vi "rad_Read FPGA Properties from INI.vi"(7 "section":string, 8 "error in (no error)":errorcluster, 11 "refnum in":T3) -> (0 "error out":errorcluster, 2 "FPGA Properties":T1=[{"Resource Name"=" ", "Path"=path ""}], 3 "refnum out":T3)   [LabVIEW 2013]
uses:
  <vilib>/Utility/config.llb/Config Data RefNum.ctl
  TypeDefs/rad_FPGA Properties.ctl
  TypeDefs/rad_FPGA Flash Properties.ctl
  <vilib>/Utility/config.llb/Read Key (I32).vi
  <vilib>/Utility/config.llb/Read Key (String).vi
  <vilib>/Utility/config.llb/NI_LVConfig.lvlib
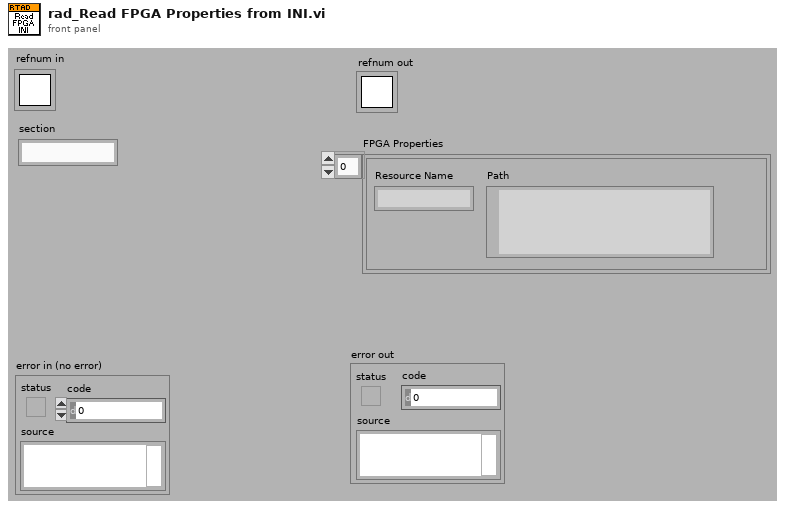
[diagram p1: front panel]
types:
  T1 = typedef "rad_FPGA Properties.ctl" = T2[]
  T2 = typedef "rad_FPGA Flash Properties.ctl" = cluster{"Resource Name":string, "Path":path}
  T3 = typedef "NI_LVConfig.lvlib/Config Data RefNum.ctl" = refnum<k1>
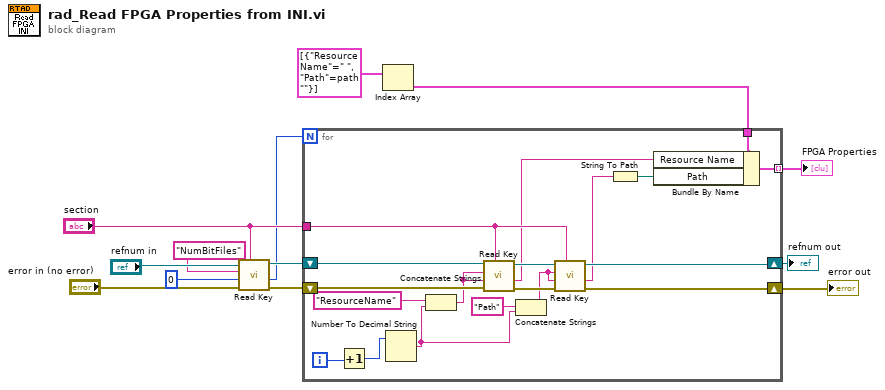
[diagram p0: block diagram]
diagram:
  n1 = call-poly <vilib>:"Read Key.vi"("section"="section", "error in (no error)"="error in (no error)", "default value"=0 ("size(s)"), "key"="NumBitFiles", "refnum"="refnum in") -> ("error out"=w7:errorcluster, "value"=w4:i32, "refnum out"=w6:T3)  [unwired: 3 in, 1 out]
  n2 = Index Array(array=T1 [{"Resource Name"=" ", "Path"=path ""}] ("FPGA Properties")) -> (element=w2:T2)  [unwired: 1 in]
  n3 = for {
    N: w4 -> [_]
    tunnel: "section" -> [w30]
    tunnel: w2 -> [w19]
    tunnel: [w14] -> w1 mode=indexing
    shift-right: [w29] -> w13
    shift-left: w6 -> [w32]
    shift-right: [w26] -> w12
    shift-left: w7 -> [w28]
    i -> [w25]
    n4 = Increment(x=w25) -> (x+1=w24:i32)
    n5 = Number To Decimal String(number=w24) -> (decimal integer string=w21:string)  [unwired: 1 in]
    n6 = Concatenate Strings("ResourceName" ("key"), w21) -> (w20:string)
    n7 = call-poly <vilib>:"Read Key.vi"("section"=w30, "error in (no error)"=w28, "default value"=w20, "key"=w20, "refnum"=w32) -> ("error out"=w27:errorcluster, "value"=w18:string, "refnum out"=w31:T3)  [unwired: 3 in, 1 out]
    n8 = Concatenate Strings("Path" ("key"), w21) -> (w17:string)
    n9 = call-poly <vilib>:"Read Key.vi"("section"=w30, "error in (no error)"=w27, "default value"=w17, "key"=w17, "refnum"=w31) -> ("error out"=w26:errorcluster, "value"=w15:string, "refnum out"=w29:T3)  [unwired: 3 in, 1 out]
    n10 = String To Path(string=w15) -> (path=w16:path)
    n11 = Bundle By Name(cluster=w19, "Resource Name"=w18, "Path"=w16) -> (w14:T2)
  }
  "error out" <- w12
  "refnum out" <- w13
  "FPGA Properties" <- w1
